vi "DEMO_06_SavePointSToMCU.vi"() -> ()   [LabVIEW 2014]
uses:
  <vilib>/Instr/_visa.llb/VISA Configure Serial Port (Instr).vi
panel:
  in  "数组个数小于48":u16
  out "发送的数组长度":i32
  in  "停止":bool
  in  "开始":bool
  out "对应Da数组的数据值":u8[](array[numeric]) format="%x"
  out "数组":dbl[](array[numeric])
  in  "设置步进时间":bool
  in  "打开串口":bool
  in  "上位机控制":bool
  in  "毫秒-0.1毫秒整数倍":dbl
  in  "存储数据到下位机":bool
  in  "通道选择":u16(ring) items=["一路", "二路", "三路"]
  in  "波特率":u32(ring)=9600 items=["75"=75, "110"=110, "134"=134, "150"=150, "300"=300, "600"=600, "1200"=1200, "1800"=1800, "2400"=2400, "4800"=4800, "7200"=7200, "9600"=9600, "14400"=14400, "19200"=19200, "28800"=28800, "38400"=38400, "56000"=56000, "57600"=57600, "115200"=115200, "128000"=128000, "230400"=230400]
  in  "奇偶":enum16{"None", "Odd", "Even", "Mark", "Space"}(ring) caption="校验"
  in  "VISA资源名称":refnum<visa-resource-name>="COM1"
  # "存储单点（多个数字信息到下位机，通过上位机设置点数以及点数的内容和发送数据时间间隔来输出任意波形数据，时间间隔为0.1豪秒的整数倍（大于0.2毫秒））"
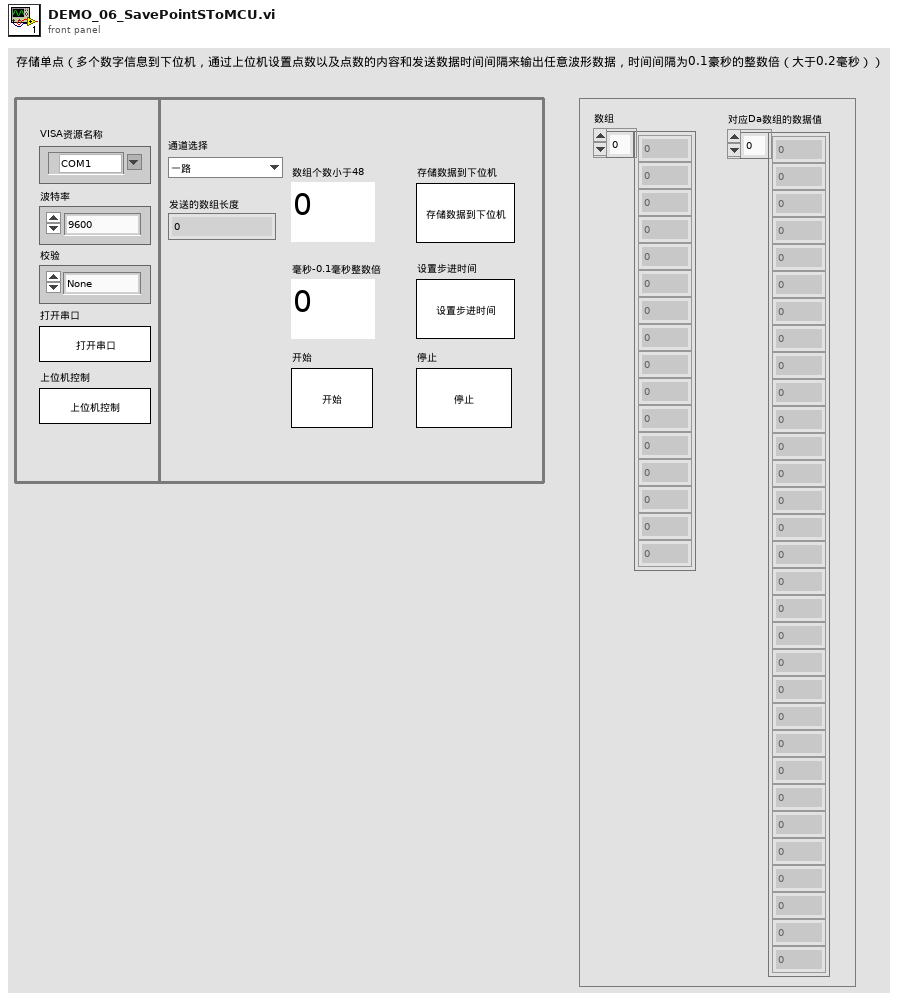
[diagram p1: front panel]
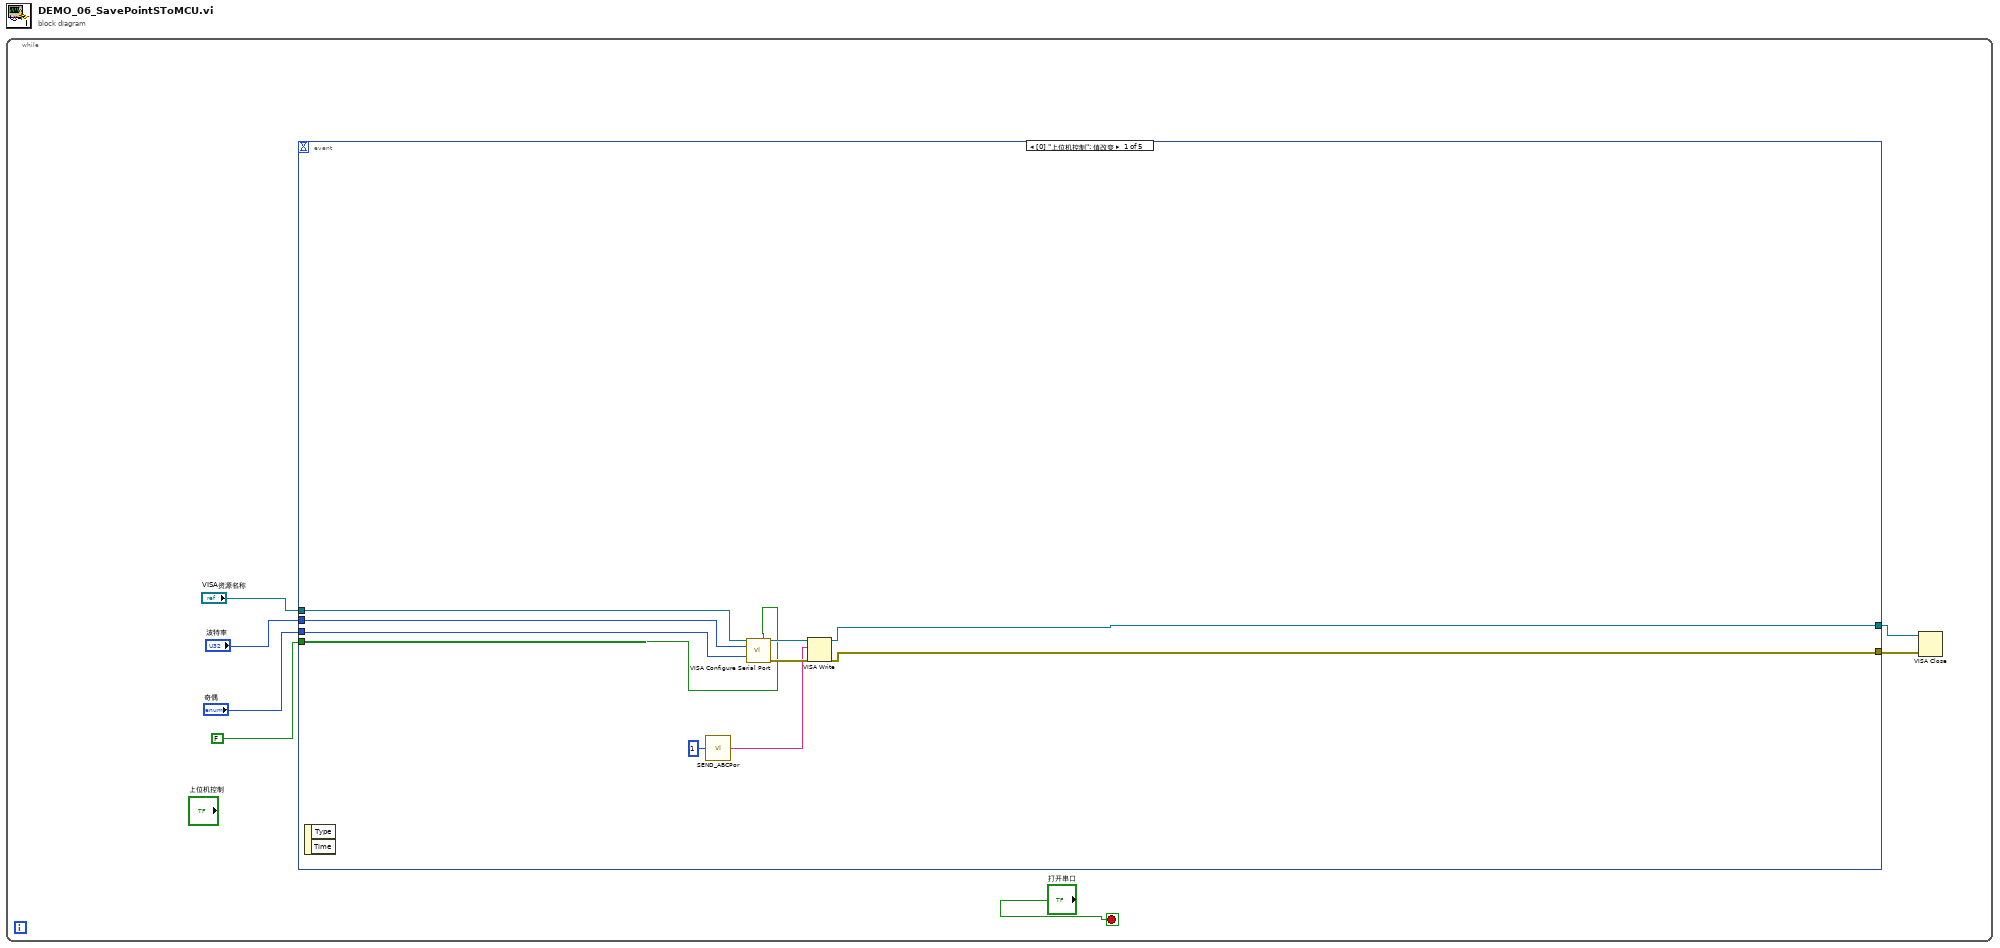
[diagram p0: block diagram]
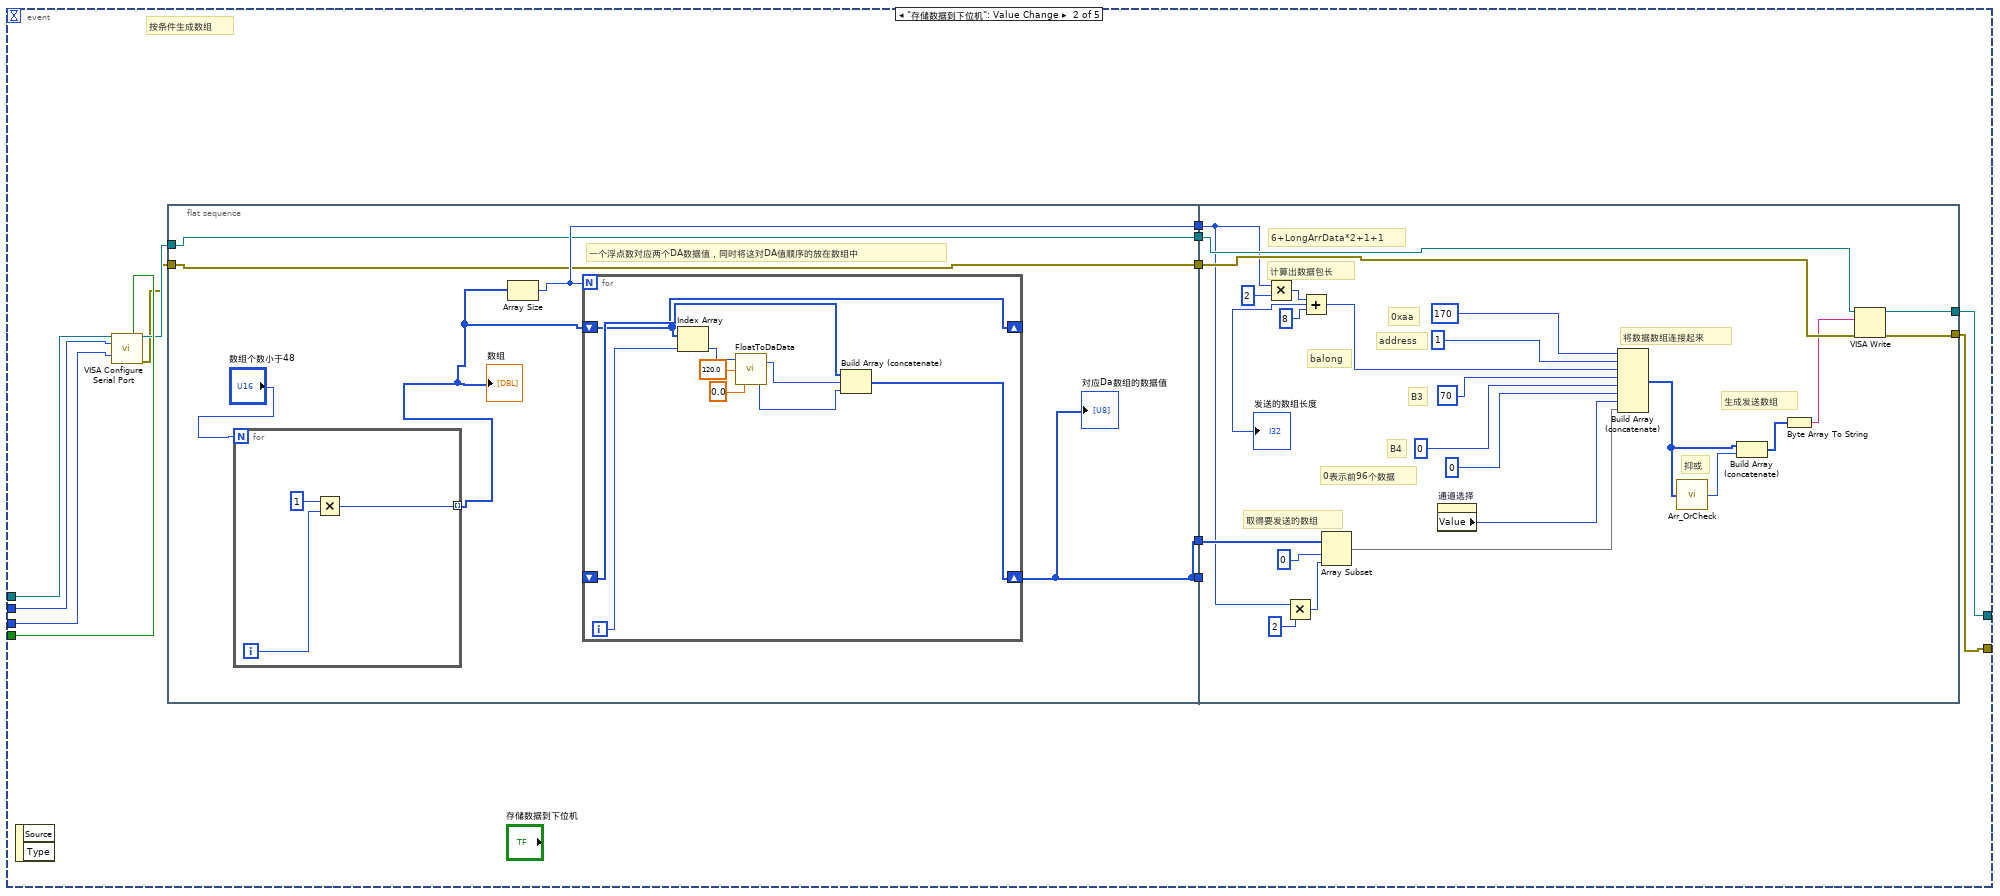
[diagram p2: hidden frame]
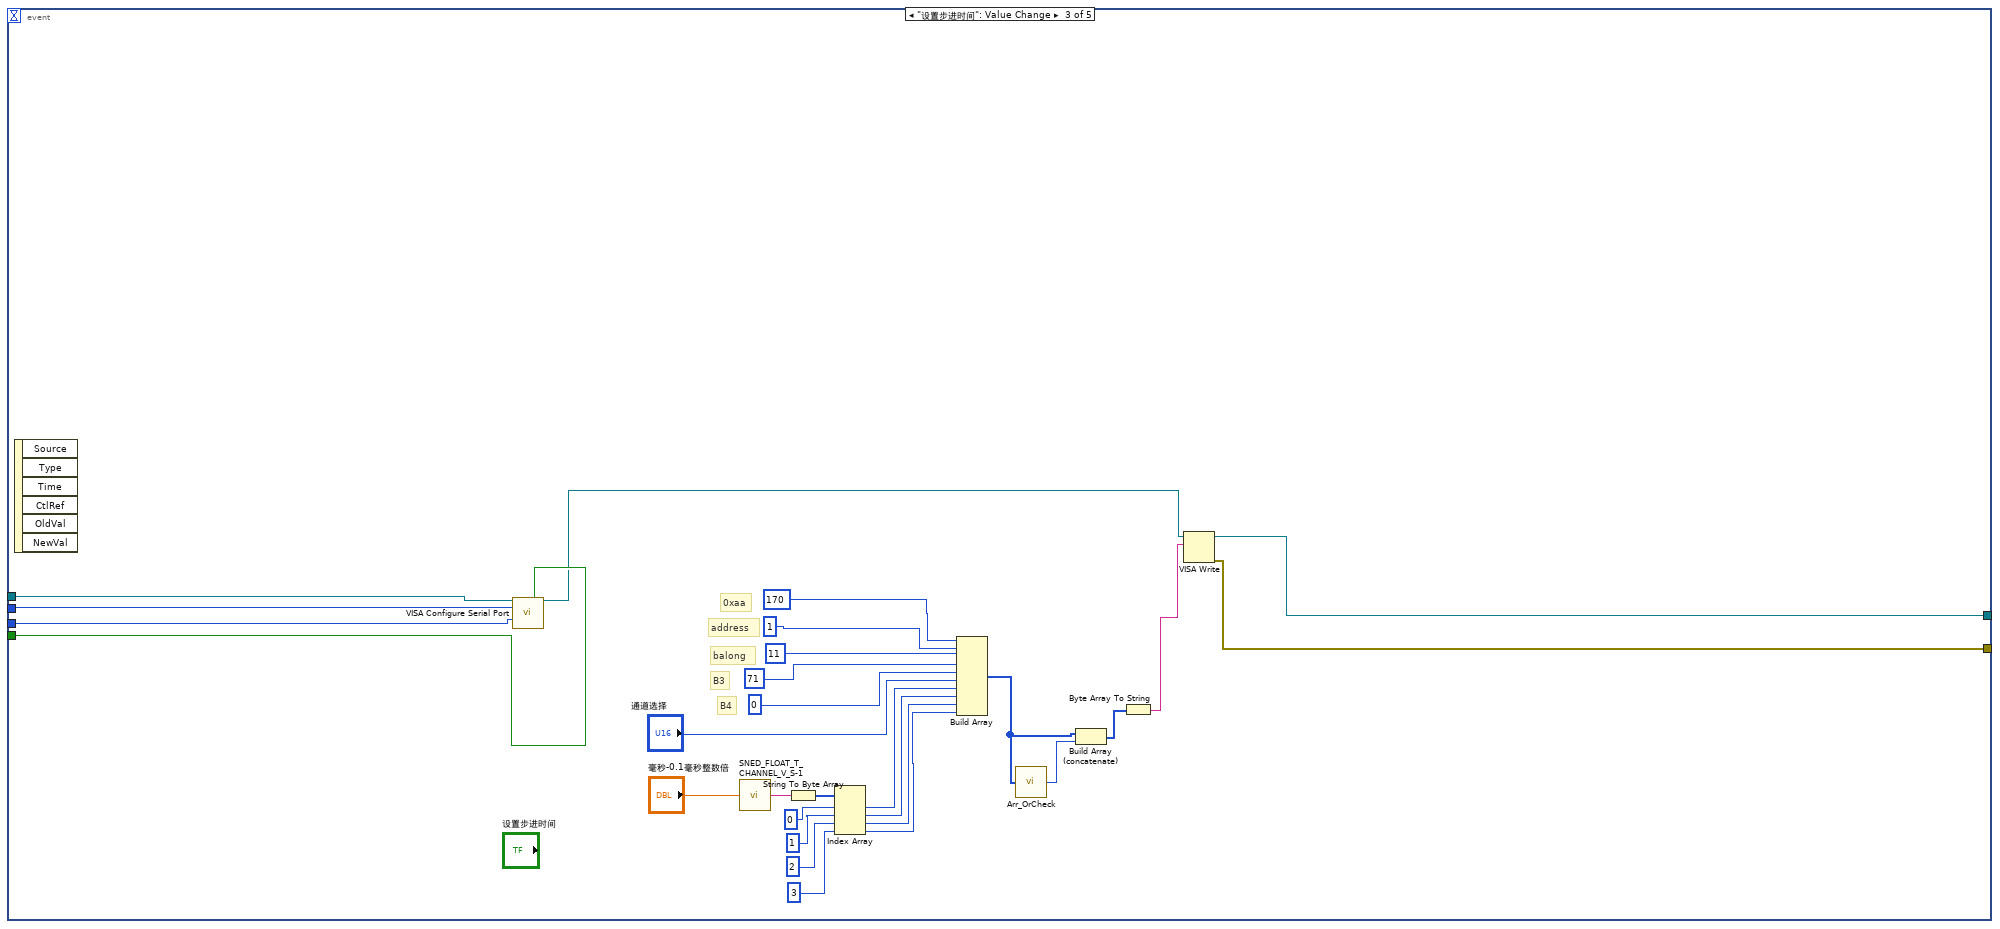
[diagram p3: hidden frame]
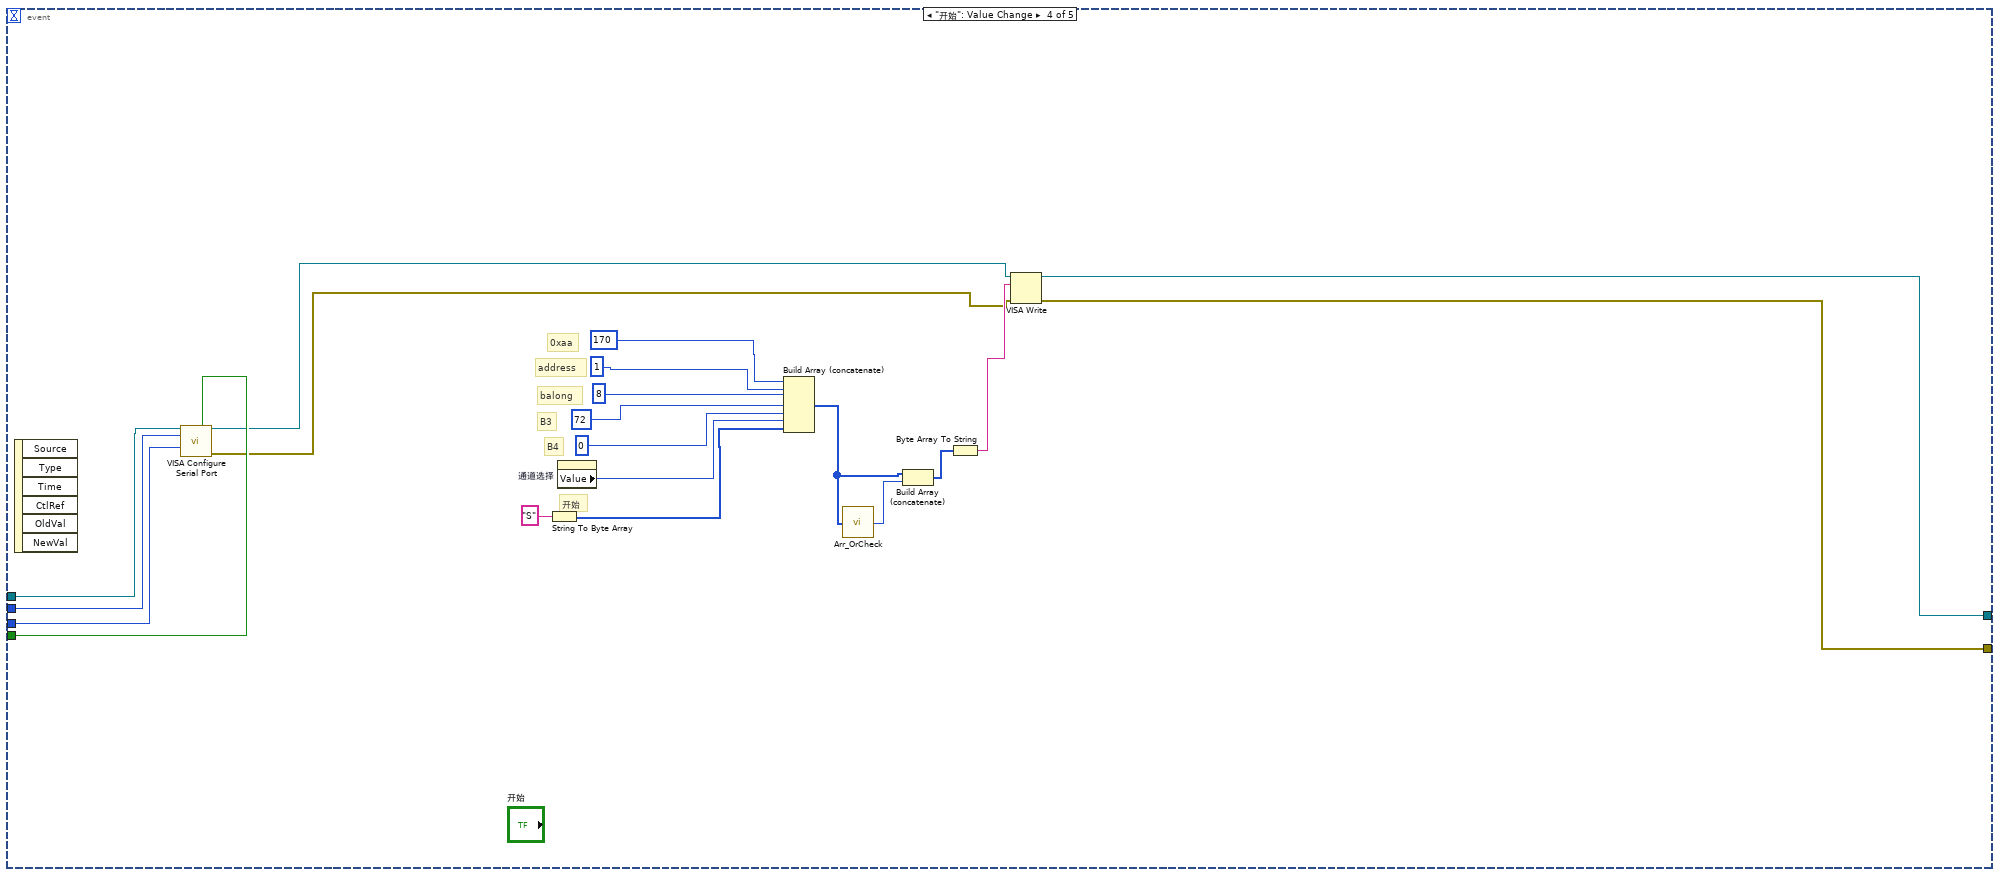
[diagram p4: hidden frame]
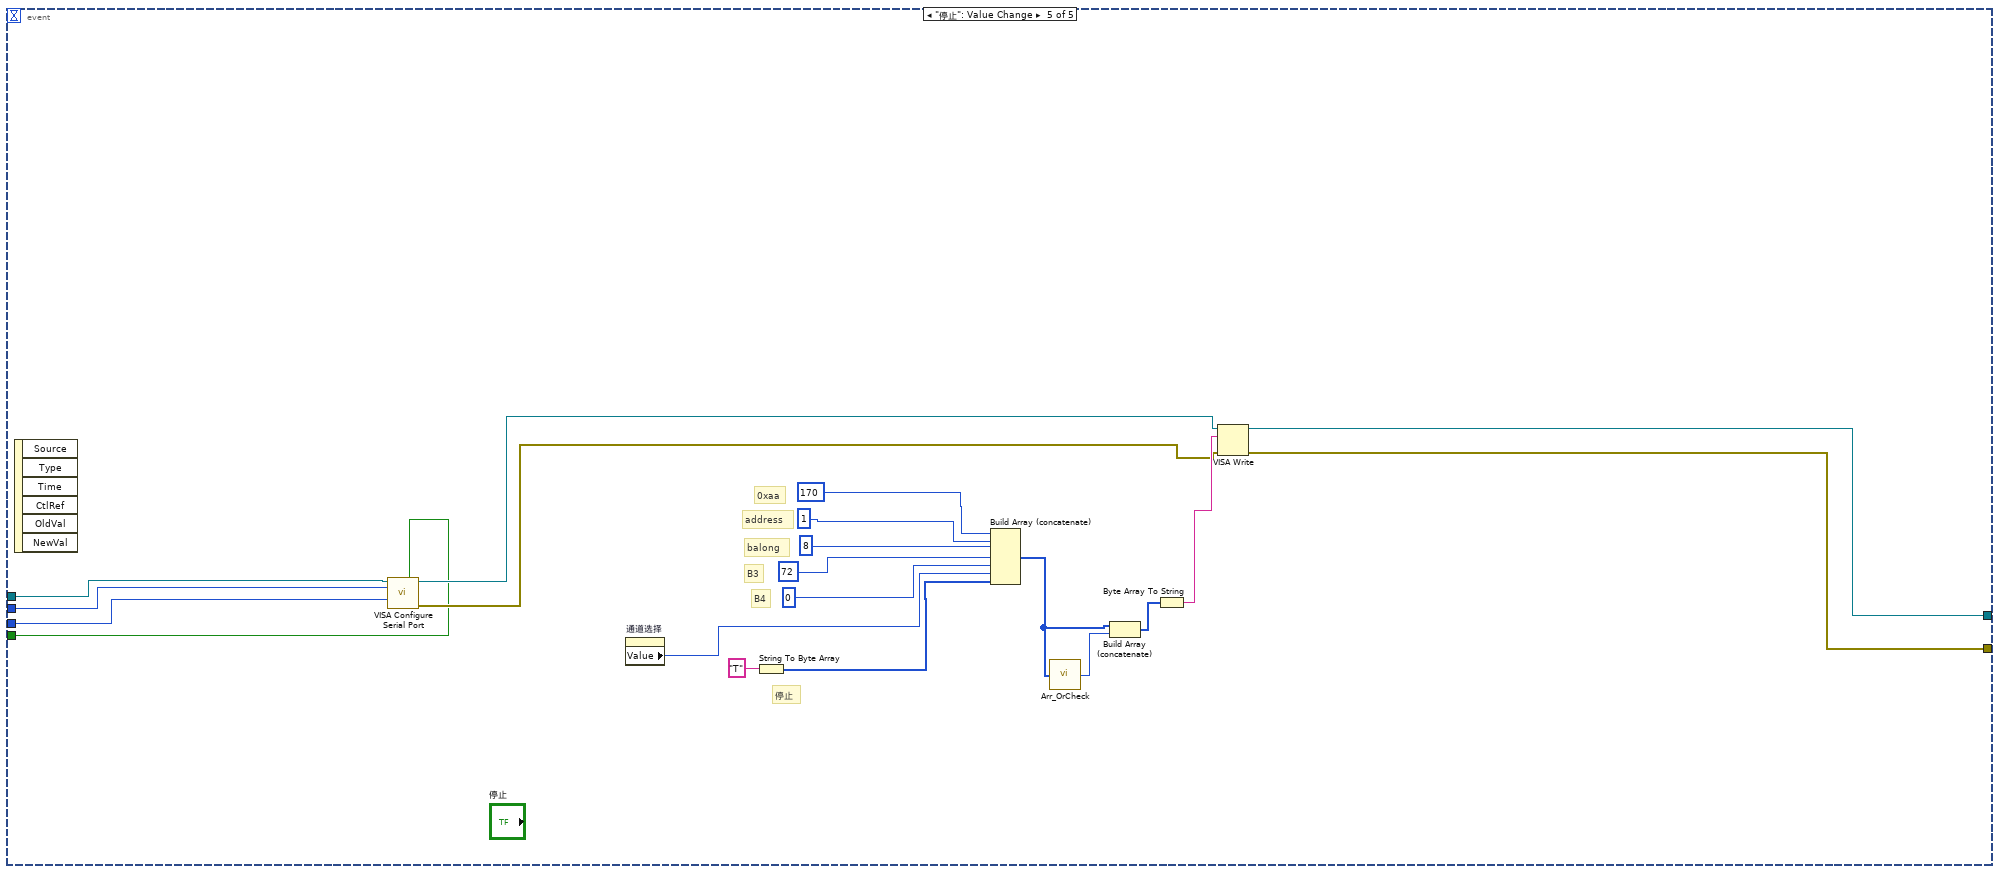
[diagram p5: hidden frame]
diagram:
  n1 = while {
    stop <- "打开串口" stop-if-true
    n2 = event shown="[0] \"上位机控制\": 值改变" {
      selector: _ -> [_ _ _ _ _]
      dyn-events: _ -> [_ _ _ _ _]
      timeout: _ -> [_ _ _ _ _]
      tunnel: [w17 w20 w73 w103 w123] -> w1
      tunnel: [w16 w19 w74 w102 w122] -> w2
      tunnel: FALSE -> [w11 w25 w100 w106 w124]
      tunnel: "VISA资源名称" -> [w8 w28 w99 w109 w127]
      tunnel: "波特率" -> [w13 w27 w98 w108 w126]
      tunnel: "奇偶" -> [w12 w26 w97 w107 w125]
      event "上位机控制": Value Change {
        n3 = event-data() -> ()  [unwired: 1 in, 2 out]
        n4 = call "SEND_ABCPor.vi"("设备地址 1 开始"=1) -> ("输出字符串"=w9:string)
        n5 = call-poly "VISA Configure Serial Port"("VISA resource name"=w8, "Enable Termination\nChar (T)"=w11, "baud rate (9600)"=w13, "parity (0:none)"=w12) -> ("VISA resource name out"=w15:refnum<visa-resource-name>, "error out"=w14:errorcluster)  [unwired: 10 in]
        n6 = VISA Write(VISA resource name=w15, write buffer=w9, error in (no error)=w14) -> (VISA resource name out=w16:refnum<visa-resource-name>, error out=w17:errorcluster)  [unwired: 1 out]
      }
      event "存储数据到下位机": Value Change {
        # "按条件生成数组"
        n7 = event-data() -> ()  [unwired: 1 in, 2 out]
        n8 = call-poly "VISA Configure Serial Port"("VISA resource name"=w28, "Enable Termination\nChar (T)"=w25, "baud rate (9600)"=w27, "parity (0:none)"=w26) -> ("VISA resource name out"=w24:refnum<visa-resource-name>, "error out"=w22:errorcluster)  [unwired: 10 in]
        n9 = flat-sequence {
          tunnel: [w36] -> w30
          tunnel: [w33] -> w29
          tunnel: w24 -> [w35]
          tunnel: [w35] -> w23
          tunnel: w22 -> [w34]
          tunnel: [w34] -> w21
          tunnel: [w33] -> w18
          tunnel: w30 -> [w52]
          tunnel: w29 -> [_]
          tunnel: w23 -> [w61]
          tunnel: w21 -> [w60]
          tunnel: [w58] -> w19
          tunnel: [w57] -> w20
          tunnel: w18 -> [w54]
          frame #0 {
            # "一个浮点数对应两个DA数据值，同时将这对DA值顺序的放在数组中"
            n10 = for {
              N: "数组个数小于48" -> [_]
              tunnel: [w37] -> w31 mode=indexing
              i -> [w38]
              n11 = Multiply(x=1, y=w38) -> (x*y=w37:i32)
            }
            "数组" <- w31
            n12 = Array Size(array=w31) -> (size(s)=w36:i32)
            n13 = for {
              N: w36 -> [_]
              shift-right: [w45] -> w33
              shift-left: _ -> [w46]
              shift-right: [w42] -> _
              shift-left: w31 -> [w42]
              i -> [w48]
              n14 = Index Array(array=w42, index=w48) -> (element=w47:i32)
              n15 = call "FloatToDaData.vi"("代表下限"=0.0, "代表上线"=120.0, "数值输入控件"=w47) -> ("x与y?-低位"=w43:u32, "floor(x/y)-高位"=w44:i16)
              n16 = Build Array (concatenate)(w46, w44, w43) -> (w45:u32[])
            }
            "对应Da数组的数据值" <- w33
          }
          frame #1 {
            # "取得要发送的数组"
            # "0表示前96个数据"
            # "计算出数据包长"
            # "生成发送数组"
            # "抑或"
            # "将数据数组连接起来"
            # "6+LongArrData*2+1+1"
            # "B4"
            # "B3"
            # "balong"
            # "address"
            # "0xaa"
            n17 = Multiply(x=w52, y=2) -> (x*y=w70:i32)
            n18 = Multiply(x=w52, y=2) -> (x*y=w50:i32)
            n19 = Add(x=w70, y=8) -> (x+y=w72:i32)
            "发送的数组长度" <- w72
            n20 = Array Subset(array=w54, index=0, length=w50) -> (w49:u32[])
            n21 = property on="通道选择" class="Ring (严格)"() -> ("Value"=w56:u16)  [unwired: 2 in, 2 out]
            n22 = Build Array (concatenate)(170, 1, w72, 70, 0, 0, w56, w49) -> (w62:u32[])
            n23 = call "Arr_OrCheck.vi"("数组"=w62) -> ("抑或的数据值"=w64:u8)
            n24 = Build Array (concatenate)(w62, w64) -> (w63:u32[])
            n25 = Byte Array To String(unsigned byte array=w63) -> (string=w59:string)
            n26 = VISA Write(VISA resource name=w61, write buffer=w59, error in (no error)=w60) -> (VISA resource name out=w58:refnum<visa-resource-name>, error out=w57:errorcluster)  [unwired: 1 out]
          }
        }
      }
      event "设置步进时间": Value Change {
        # "B4"
        # "B3"
        # "balong"
        # "address"
        # "0xaa"
        n27 = event-data() -> ()  [unwired: 1 in, 6 out]
        n28 = call-poly "VISA Configure Serial Port"("VISA resource name"=w99, "Enable Termination\nChar (T)"=w100, "baud rate (9600)"=w98, "parity (0:none)"=w97) -> ("VISA resource name out"=w75:refnum<visa-resource-name>)  [unwired: 10 in, 1 out]
        n29 = call "SNED_FLOAT_T_CHANNEL_V_S-1.vi"("数据"="毫秒-0.1毫秒整数倍") -> ("字符串"=w96:string)
        n30 = String To Byte Array(string=w96) -> (unsigned byte array=w95:u8[])
        n31 = Index Array(array=w95, index #1=0, index #2=1, index #3=2, index #4=3) -> (element #1=w83:u8, element #2=w82:u8, element #3=w81:u8, element #4=w80:u8)
        n32 = Build Array(170, 1, 11, 71, 0, "通道选择", w83, w82, w81, w80) -> (w79:i32[])
        n33 = call "Arr_OrCheck.vi"("数组"=w79) -> ("抑或的数据值"=w90:u8)
        n34 = Build Array (concatenate)(w79, w90) -> (w89:i32[])
        n35 = Byte Array To String(unsigned byte array=w89) -> (string=w88:string)
        n36 = VISA Write(VISA resource name=w75, write buffer=w88) -> (VISA resource name out=w74:refnum<visa-resource-name>, error out=w73:errorcluster)  [unwired: 1 in, 1 out]
      }
      event "开始": Value Change {
        # "开始"
        # "B4"
        # "B3"
        # "balong"
        # "address"
        # "0xaa"
        n37 = event-data() -> ()  [unwired: 1 in, 6 out]
        n38 = call-poly "VISA Configure Serial Port"("VISA resource name"=w109, "Enable Termination\nChar (T)"=w106, "baud rate (9600)"=w108, "parity (0:none)"=w107) -> ("VISA resource name out"=w105:refnum<visa-resource-name>, "error out"=w104:errorcluster)  [unwired: 10 in]
        n39 = String To Byte Array(string="S") -> (unsigned byte array=w110:u8[])
        n40 = property on="通道选择" class="Ring (严格)"() -> ("Value"=w101:u16)  [unwired: 2 in, 2 out]
        n41 = Build Array (concatenate)(170, 1, 8, 72, 0, w101, w110) -> (w113:i32[])
        n42 = call "Arr_OrCheck.vi"("数组"=w113) -> ("抑或的数据值"=w120:u8)
        n43 = Build Array (concatenate)(w113, w120) -> (w119:i32[])
        n44 = Byte Array To String(unsigned byte array=w119) -> (string=w118:string)
        n45 = VISA Write(VISA resource name=w105, write buffer=w118, error in (no error)=w104) -> (VISA resource name out=w102:refnum<visa-resource-name>, error out=w103:errorcluster)  [unwired: 1 out]
      }
      event "停止": Value Change {
        # "停止"
        # "B4"
        # "B3"
        # "balong"
        # "address"
        # "0xaa"
        n46 = event-data() -> ()  [unwired: 1 in, 6 out]
        n47 = call-poly "VISA Configure Serial Port"("VISA resource name"=w127, "Enable Termination\nChar (T)"=w124, "baud rate (9600)"=w126, "parity (0:none)"=w125) -> ("VISA resource name out"=w129:refnum<visa-resource-name>, "error out"=w128:errorcluster)  [unwired: 10 in]
        n48 = property on="通道选择" class="Ring (严格)"() -> ("Value"=w121:u16)  [unwired: 2 in, 2 out]
        n49 = String To Byte Array(string="T") -> (unsigned byte array=w130:u8[])
        n50 = Build Array (concatenate)(170, 1, 8, 72, 0, w121, w130) -> (w133:i32[])
        n51 = call "Arr_OrCheck.vi"("数组"=w133) -> ("抑或的数据值"=w140:u8)
        n52 = Build Array (concatenate)(w133, w140) -> (w139:i32[])
        n53 = Byte Array To String(unsigned byte array=w139) -> (string=w138:string)
        n54 = VISA Write(VISA resource name=w129, write buffer=w138, error in (no error)=w128) -> (VISA resource name out=w122:refnum<visa-resource-name>, error out=w123:errorcluster)  [unwired: 1 out]
      }
    }
    n55 = VISA Close(VISA resource name=w2, error in (no error)=w1) -> ()  [unwired: 1 out]
  }
